vi "AMWave.vi"(2 "AM Wave Parameters":T1, 3 "Digitizing Parameters":T2) -> (0 "AM Wave":cluster{"Time":dbl[], "Displacement":dbl[]}, 1 "XY Graph":cluster{"t":dbl[], "x":dbl[]}(graph))   [LabVIEW 2015]
uses:
  <vilib>/imath/engines/lvmath2/RunTimeEngine/Managers/WorkSpace/UID Generator.vi
  <vilib>/imath/engines/lvmath2/RunTimeEngine/RunTimeType/NIMS_RunTimeType_From StrictType (excl LVString).vi
  <instcachedir>/0/NIMS_RunTimeType_From StrictType (excl LVString)_EB1C38A9BC5048DA9ABDA8F781E54D21.lvgen/NIMS_RunTimeType_From StrictType (excl LVString)_EB1C38A9BC5048DA9ABDA8F781E54D21_000.vi
  <vilib>/imath/engines/lvmath2/RunTimeEngine/LocalVariableDefStatement/MC_LocalVariableDefStatement_Display.vi
  <vilib>/imath/engines/lvmath2/RunTimeEngine/RangeToken/NIMS_Range.vi
  <instcachedir>/0/NIMS_Range_D919CC09935940E88F755EC1C6F49AC1.lvgen/NIMS_Range_D919CC09935940E88F755EC1C6F49AC1_000.vi
  <vilib>/imathl/engines/lvmath/Functions/Error Handling/Create Error.vi
  <vilib>/imath/engines/lvmath2/RunTimeEngine/ArithmeticOperatorToken/NIMS_ArithmeticOperator_times.vi
  <instcachedir>/0/NIMS_ArithmeticOperator_times_DF26C4080E2A467BA28C929B8CF31953.lvgen/NIMS_ArithmeticOperator_times_DF26C4080E2A467BA28C929B8CF31953_000.vi
  <vilib>/imath/engines/lvmath2/RunTimeEngine/Managers/SymbolTable/Clear UID.vi
  <vilib>/imath/engines/lvmath2/RunTimeEngine/NodeEndStatement/NIMS_NodeEndStatement_Output.vi
  <instcachedir>/0/NIMS_NodeEndStatement_Output_53EC0D466D134D7ABD903AC30B43404B.lvgen/NIMS_NodeEndStatement_Output_53EC0D466D134D7ABD903AC30B43404B_005.vi
  <vilib>/imath/engines/lvmath2/RunTimeEngine/ErrorHandling/NIMS_Finalize Error.vi
  <vilib>/imath/engines/lvmath2/RunTimeEngine/Managers/SymbolTable/NIMS_WorkSpace.lvlib
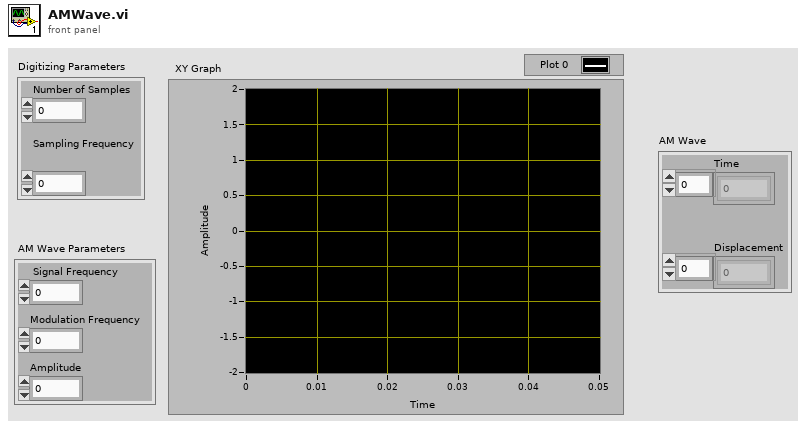
[diagram p1: front panel]
types:
  T1 = cluster{" Signal Frequency":dbl, "Modulation Frequency":dbl, "Amplitude":dbl}
  T2 = cluster{"Number of Samples":dbl, "Sampling Frequency":dbl}
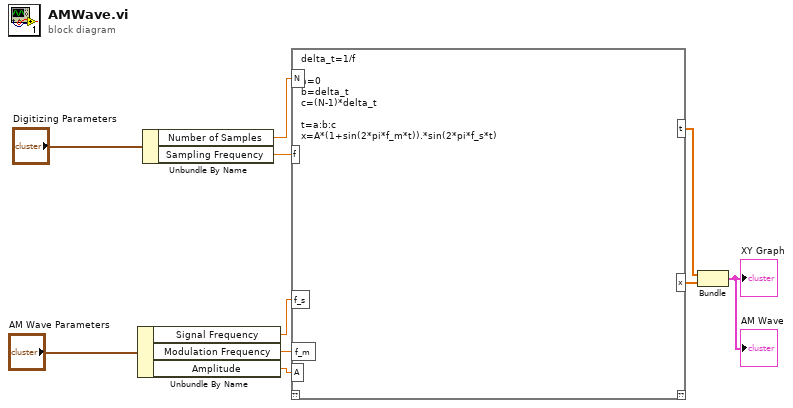
[diagram p0: block diagram]
diagram:
  n1 = Unbundle By Name("AM Wave Parameters") -> ("Signal Frequency"=w3:dbl, "Modulation Frequency"=w2:dbl, "Amplitude"=w1:dbl)
  n2 = Unbundle By Name("Digitizing Parameters") -> ("Number of Samples"=w5:dbl, "Sampling Frequency"=w4:dbl)
  n3 = mathscript code="delta_t=1/f\n\na=0\nb=delta_t\nc=(N-1)*delta_t\n\nt=a:b:c\nx=A*(1+sin(2*pi*f_m*t)).*sin(2*pi*f_s*t)"("N"=w5, "f"=w4, "f_s"=w3, "f_m"=w2, "A"=w1) -> ("t"=w9:dbl[], "x"=w10:dbl[])  [unwired: 1 in, 1 out]
  n4 = Bundle("t"=w9, "x"=w10) -> (→"XY Graph" →"AM Wave":cluster{"t":dbl[], "x":dbl[]})  [unwired: 1 in]
